vi "TDT-Get All Events.vi"(0 "Data":T1={"TTankX"=refnum, "TDevAccX"=refnum, "LastTime"=0.0, "error"={"status"=FALSE, "code"=0, "source"=""}, "Block Name"="", "Circuit Tag"="", "Tank Name"="", "NumTicks"=0, "LastTick"=0.0, "Idle?"=FALSE, "Wait (ms)"=1000, "LastArtf"=0.0, "LastTosc"=0.0}, 7 "Max Read":i32=20000, 11 "error in (no error)":errorcluster) -> (8 "Events":dbl[][](array[numeric]), 15 "error out":errorcluster)   [LabVIEW 2015]
uses:
  TDT Interface Data.ctl
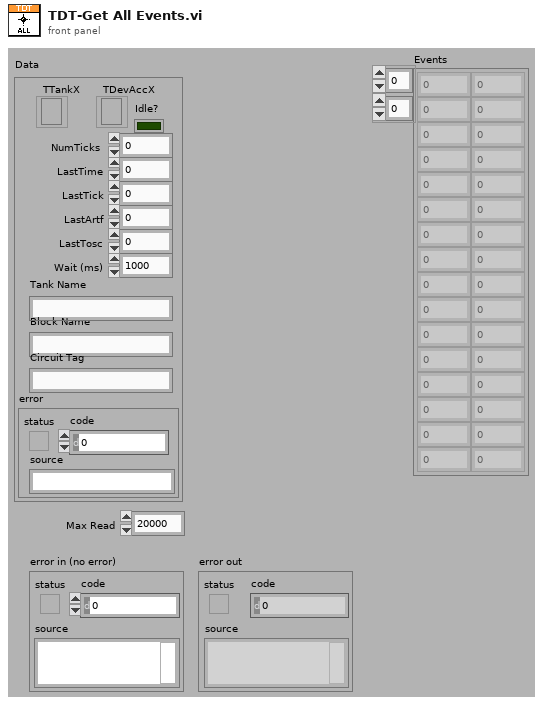
[diagram p1: front panel]
types:
  T1 = typedef "TDT Interface Data.ctl" = cluster{"TTankX":refnum<k7>, "TDevAccX":refnum<k7>, "LastTime":dbl, "error":errorcluster, "Block Name":string, "Circuit Tag":string, "Tank Name":string, "NumTicks":i32, "LastTick":dbl, "Idle?":bool, "Wait (ms)":u32, "LastArtf":dbl, "LastTosc":dbl}
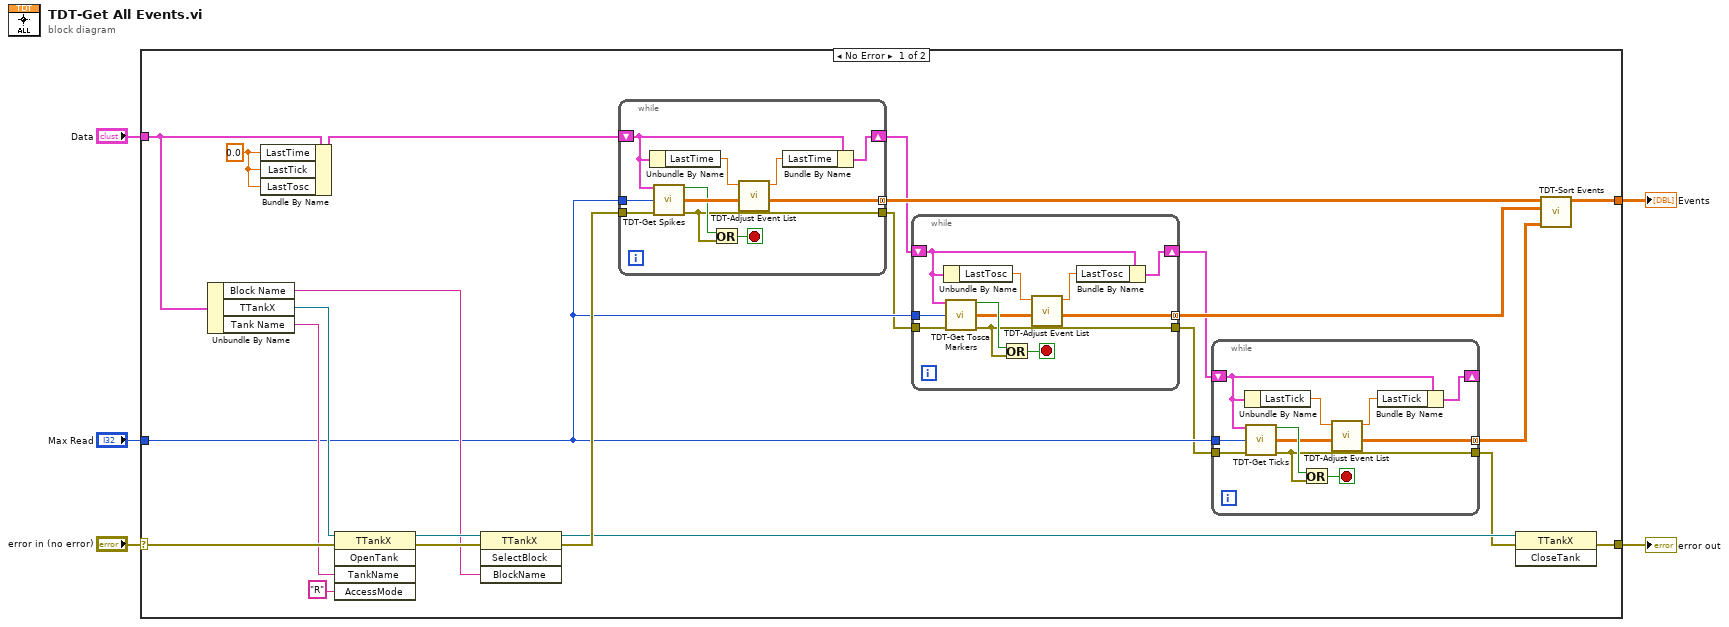
[diagram p0: block diagram]
diagram:
  n1 = case shown="No Error" "error in (no error)" {
    selector: "error in (no error)" -> [w25 w62]
    tunnel: [w24 w62] -> w4
    tunnel: "Data" -> [w18 _]
    tunnel: "Max Read" -> [w13 _]
    tunnel: [w28 _] -> w1
    frame No Error {
      w14 = 0.0 ("LastTime")
      n2 = Unbundle By Name(w18) -> ("Block Name"=w20:string, "TTankX"=w17:refnum<k7>, "Tank Name"=w21:string)
      n3 = Bundle By Name(cluster=w18, "LastTime"=w14, "LastTick"=w14, "LastTosc"=w14) -> (w16:T1)
      n4 = invoke class="TTankX" method="OpenTank"(reference=w17, error in=w25, "TankName"=w21, "AccessMode"="R") -> (reference out=w22:refnum<k7>, error out=w23:errorcluster)  [unwired: 1 in, 3 out]
      n5 = invoke class="TTankX" method="SelectBlock"(reference=w22, error in=w23, "BlockName"=w20) -> (reference out=w8:refnum<k7>, error out=w26:errorcluster)  [unwired: 1 in, 2 out]
      n6 = while {
        tunnel: [w40] -> w9
        tunnel: [w49] -> w27 mode=concatenating
        tunnel: w26 -> [w48]
        tunnel: w13 -> [w47]
        shift-right: [w43] -> w10
        shift-left: w16 -> [w45]
        stop <- w41 stop-if-true
        n7 = Unbundle By Name(w45) -> ("LastTime"=w46:dbl)
        n8 = call "TDT-Get Spikes.vi"("Data"=w45, "Max Read"=w47, "error in (no error)"=w48) -> ("Got 'em all"=w42:bool, "Spike times"=w50:dbl[][], "error out"=w40:errorcluster)  [unwired: 9 in, 1 out]
        n9 = Or(x=w42, y=w40) -> (x .or. y?=w41:bool)
        n10 = call "TDT-Adjust Event List.vi"("Events in"=w50, "Last In"=w46) -> ("Events out"=w49:dbl[][], "Last out"=w44:dbl)  [unwired: 8 in]
        n11 = Bundle By Name(cluster=w45, "LastTime"=w44) -> (w43:T1)
      }
      n12 = while {
        tunnel: [w39] -> w15 mode=concatenating
        tunnel: w9 -> [w35]
        tunnel: w13 -> [w34]
        shift-right: [w36] -> w12
        shift-left: w10 -> [w33]
        tunnel: [w29] -> w7
        stop <- w30 stop-if-true
        n13 = Unbundle By Name(w33) -> ("LastTosc"=w38:dbl)
        n14 = call "TDT-Get Tosca Markers.vi"("Data"=w33, "Max Read"=w34, "error in (no error)"=w35) -> ("Got em' all"=w32:bool, "Tosca markers"=w31:dbl[][], "error out"=w29:errorcluster)  [unwired: 10 in]
        n15 = Or(x=w32, y=w29) -> (x .or. y?=w30:bool)
        n16 = call "TDT-Adjust Event List.vi"("Events in"=w31, "Last In"=w38) -> ("Events out"=w39:dbl[][], "Last out"=w37:dbl)  [unwired: 8 in]
        n17 = Bundle By Name(cluster=w33, "LastTosc"=w37) -> (w36:T1)
      }
      n18 = while {
        tunnel: [w61] -> w11 mode=concatenating
        tunnel: w7 -> [w57]
        tunnel: w13 -> [w56]
        shift-right: [w58] -> _
        shift-left: w12 -> [w55]
        tunnel: [w51] -> w6
        stop <- w52 stop-if-true
        n19 = Unbundle By Name(w55) -> ("LastTick"=w60:dbl)
        n20 = call "TDT-Get Ticks.vi"("Data"=w55, "Max Read"=w56, "error in (no error)"=w57) -> ("Got 'em all"=w54:bool, "Tick times"=w53:dbl[][], "error out"=w51:errorcluster)  [unwired: 9 in, 1 out]
        n21 = Or(x=w54, y=w51) -> (x .or. y?=w52:bool)
        n22 = call "TDT-Adjust Event List.vi"("Events in"=w53, "Last In"=w60) -> ("Events out"=w61:dbl[][], "Last out"=w59:dbl)  [unwired: 8 in]
        n23 = Bundle By Name(cluster=w55, "LastTick"=w59) -> (w58:T1)
      }
      n24 = invoke class="TTankX" method="CloseTank"(reference=w8, error in=w6) -> (error out=w24:errorcluster)  [unwired: 1 in, 2 out]
      n25 = call "TDT-Sort Events.vi"("Tosca Markers"=w11, "Spikes"=w15, "Ticks"=w27) -> ("Sorted events"=w28:dbl[][])  [unwired: 8 in]
    }
    frame Error {
    }
  }
  "error out" <- w4
  "Events" <- w1
